vi "Get Statistics.vi"(11 "Result Model in":refnum<class "Result Model.lvclass">) -> (2 "Results":T1)   [LabVIEW 2020, in "Result Model.lvclass"]
uses:
  Result Model.lvclass
  Statistics.ctl
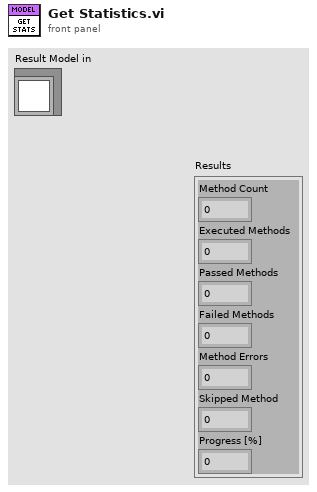
[diagram p1: front panel]
types:
  T1 = typedef "Result Model.lvclass/Statistics.ctl" = cluster{"Method Count":u32, "Executed Methods":u32, "Passed Methods":u32, "Failed Methods":u32, "Method Errors":u32, "Skipped Method":u32, "Progress [%]":dbl}
  T2 = typedef "Result.lvlib/Status.ctl" = enum16{"", "Passed", "Failed", "Error", "Skipped", "Setup Error", "Broken", "Teardown Error"}
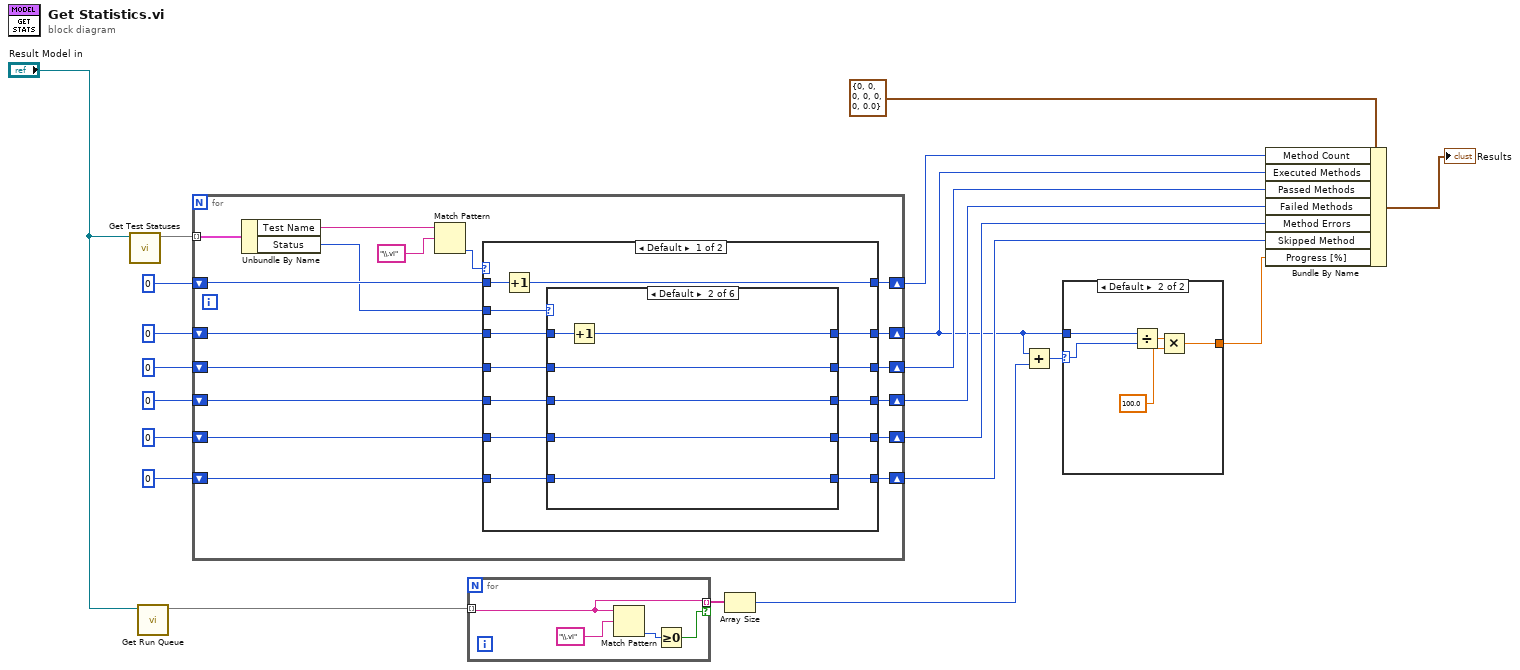
[diagram p0: block diagram]
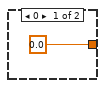
[diagram p2: hidden frame]
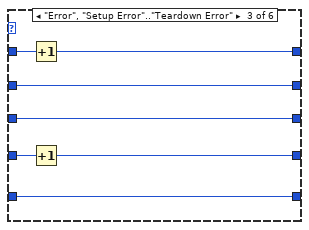
[diagram p4: hidden frame]
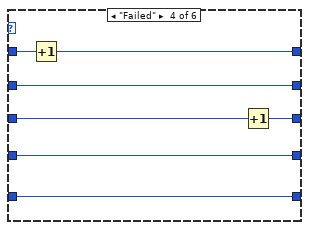
[diagram p5: hidden frame]
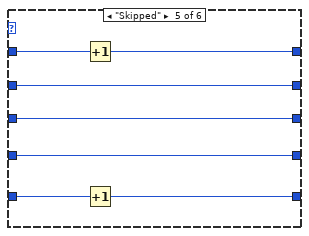
[diagram p6: hidden frame]
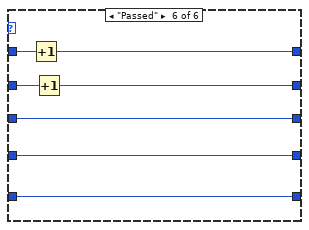
[diagram p7: hidden frame]
diagram:
  n1 = call "Get Test Statuses.vi"("Result Model in"="Result Model in") -> ("Test Statuses"=w3:map{string, T2})  [unwired: 10 in]
  n2 = call "Get Run Queue.vi"("Result Model in"="Result Model in") -> ("Run Queue"=w1:set{string})  [unwired: 10 in]
  n3 = for {
    tunnel: w3 -> [w38] mode=indexing
    shift-right: [w33] -> w9
    shift-left: u32 0 ("Method Count") -> [w34]
    shift-right: [w30] -> w7
    shift-left: u32 0 ("Method Count") -> [w31]
    shift-right: [w28] -> w17
    shift-left: u32 0 ("Method Count") -> [w29]
    shift-right: [w26] -> w15
    shift-left: u32 0 ("Method Count") -> [w27]
    shift-right: [w24] -> w13
    shift-left: u32 0 ("Method Count") -> [w25]
    shift-right: [w22] -> w11
    shift-left: u32 0 ("Method Count") -> [w23]
    n4 = Unbundle By Name(w38) -> ("Test Name"=w37:string, "Status"=w32:T2)
    n5 = Match Pattern(string=w37, regular expression="\\.vi") -> (offset past match=w35:i32)  [unwired: 1 in, 3 out]
    n6 = case shown="Default" w35 {
      tunnel: w34 -> [w51 w96]
      tunnel: [w50 w96] -> w33
      tunnel: w32 -> [w49 _]
      tunnel: w31 -> [w48 w95]
      tunnel: [w47 w95] -> w30
      tunnel: w29 -> [w46 w94]
      tunnel: [w45 w94] -> w28
      tunnel: w27 -> [w44 w93]
      tunnel: [w43 w93] -> w26
      tunnel: w25 -> [w42 w92]
      tunnel: [w41 w92] -> w24
      tunnel: w23 -> [w40 w91]
      tunnel: [w39 w91] -> w22
      frame Default {
        n7 = Increment(x=w51) -> (x+1=w50:u32)
        n8 = case shown="Default" w49 {
          tunnel: w48 -> [w56 w62 w69 w76 w83 w90]
          tunnel: [w56 w61 w68 w75 w82 w89] -> w47
          tunnel: w46 -> [w55 w60 w67 w74 w81 w88]
          tunnel: [w55 w60 w67 w74 w81 w87] -> w45
          tunnel: w44 -> [w54 w59 w66 w73 w80 w86]
          tunnel: [w54 w59 w66 w72 w80 w86] -> w43
          tunnel: w42 -> [w53 w58 w65 w71 w79 w85]
          tunnel: [w53 w58 w64 w71 w79 w85] -> w41
          tunnel: w40 -> [w52 w57 w63 w70 w78 w84]
          tunnel: [w52 w57 w63 w70 w77 w84] -> w39
          frame "" {
          }
          frame Default {
            n9 = Increment(x=w62) -> (x+1=w61:u32)
          }
          frame "Error", "Setup Error".."Teardown Error" {
            n10 = Increment(x=w69) -> (x+1=w68:u32)
            n11 = Increment(x=w65) -> (x+1=w64:u32)
          }
          frame "Failed" {
            n12 = Increment(x=w76) -> (x+1=w75:u32)
            n13 = Increment(x=w73) -> (x+1=w72:u32)
          }
          frame "Skipped" {
            n14 = Increment(x=w83) -> (x+1=w82:u32)
            n15 = Increment(x=w78) -> (x+1=w77:u32)
          }
          frame "Passed" {
            n16 = Increment(x=w90) -> (x+1=w89:u32)
            n17 = Increment(x=w88) -> (x+1=w87:u32)
          }
        }
      }
      frame -1 {
      }
    }
  }
  n18 = for {
    tunnel: w1 -> [w98] mode=indexing
    tunnel: [w98] -> w5 mode=indexing if=w97
    n19 = Match Pattern(string=w98, regular expression="\\.vi") -> (offset past match=w99:i32)  [unwired: 1 in, 3 out]
    n20 = Greater Or Equal To 0?(x=w99) -> (x >= 0?=w97:bool)
  }
  n21 = Array Size(array=w5) -> (size(s)=w4:i32)
  n22 = Add(x=w7, y=w4) -> (x+y=w6:u32)
  n23 = case shown="Default" w6 {
    selector: w6 -> [_ w102]
    tunnel: w7 -> [_ w103]
    tunnel: [0.0 w104] -> w8
    frame 0 {
    }
    frame Default {
      n24 = Divide(x=w103, y=w102) -> (x/y=w106:dbl)
      n25 = Multiply(x=w106, y=100.0) -> (x*y=w104:dbl)
    }
  }
  n26 = Bundle By Name(cluster=T1 {"Method Count"=0, "Executed Methods"=0, "Passed Methods"=0, "Failed Methods"=0, "Method Errors"=0, "Skipped Method"=0, "Progress [%]"=0.0} ("Results"), "Method Count"=w9, "Executed Methods"=w7, "Passed Methods"=w17, "Failed Methods"=w15, "Method Errors"=w13, "Skipped Method"=w11, "Progress [%]"=w8) -> (→"Results":T1)
